vi "(Un)register Error Status Callback.vi"(7 "Unregister? [F, register]":bool, 10 "Arr Refnum [NOP]":refnum<vi>) -> (2 "Registered controls":refnum<vi>[](array[refnum]))   [LabVIEW 2020, in "Multiple Errors.lvclass"]
uses:
  Multiple Errors.lvclass
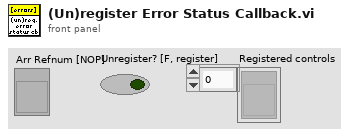
[diagram p1: front panel]
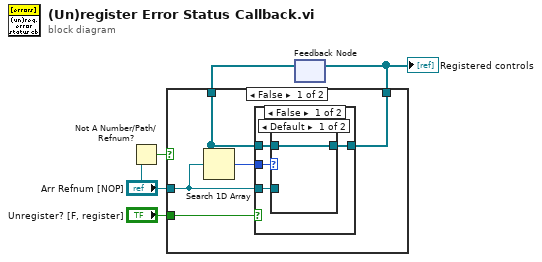
[diagram p0: block diagram]
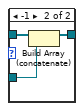
[diagram p2: hidden frame]
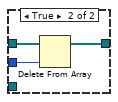
[diagram p3: hidden frame]
diagram:
  n1 = Not A Number/Path/Refnum?(number/path/refnum="Arr Refnum [NOP]") -> (NaN/Path/Refnum?=w1:bool)
  n2 = feedback #1() -> (w4:refnum<vi>[])  [unwired: 1 in]
  n3 = case shown="False" w1 {
    tunnel: "Unregister? [F, register]" -> [w10 _]
    tunnel: w4 -> [w9 w22]
    tunnel: "Arr Refnum [NOP]" -> [w7 _]
    tunnel: [w6 w22] -> w3
    frame False {
      n4 = Search 1D Array(1D array=w9, element=w7) -> (index of element=w8:i32)  [unwired: 1 in]
      n5 = case shown="False" w10 {
        tunnel: w9 -> [w13 w21]
        tunnel: w8 -> [w14 w20]
        tunnel: [w11 w19] -> w6
        tunnel: w7 -> [w12 _]
        frame False {
          n6 = case shown="Default" w14 {
            tunnel: w13 -> [w15 w18]
            tunnel: w12 -> [_ w17]
            tunnel: [w15 w16] -> w11
            frame Default {
            }
            frame -1 {
              n7 = Build Array (concatenate)(w18, w17) -> (w16:refnum<vi>[])
            }
          }
        }
        frame True {
          n8 = Delete From Array(array=w21, index=w20) -> (array with subset deleted=w19:refnum<vi>[])  [unwired: 1 in, 1 out]
        }
      }
    }
    frame True {
    }
  }
  "Registered controls" <- w3
  n9 = feedback-in #1(w3) -> ()
